vi "ReleaseBufferAndRemove.vi"(7 "index":i32, 8 "error in (no error)":errorcluster, 9 "pointer":u64, 10 "Buffer Name":string, 11 "Buffers":T1[](array[typedef])) -> (0 "error out":errorcluster, 2 "output buffer":T1, 3 "output buffers":T1[](array[typedef]))   [LabVIEW 2016]
uses:
  private/vis/BufferStruct.ctl
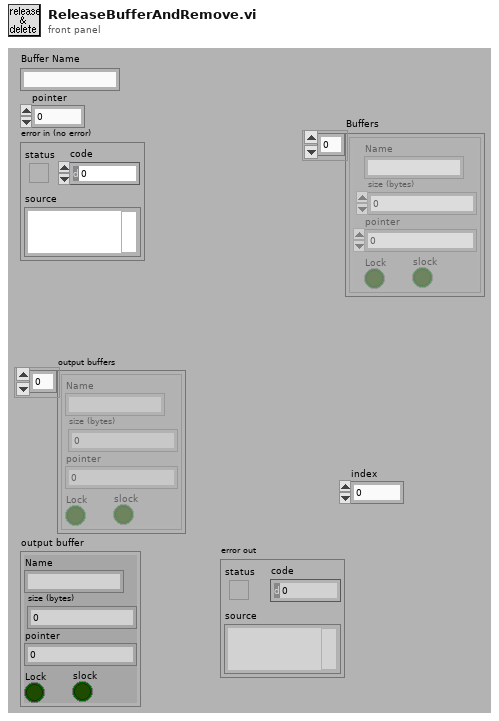
[diagram p1: front panel]
types:
  T1 = typedef "BufferStruct.ctl" = cluster{"Name":string, "size (bytes)":u64, "pointer":u64, "Lock":bool, "slock":bool}
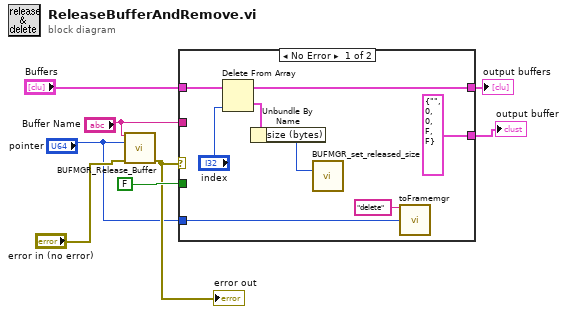
[diagram p0: block diagram]
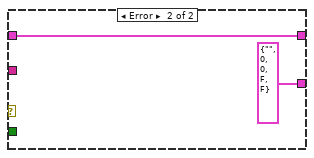
[diagram p2: hidden frame]
diagram:
  n1 = call "BUFMGR_Release_Buffer.vi"("Buffer Name"="Buffer Name", "buffer in"="pointer", "error in (no error)"="error in (no error)") -> ("error out"=w3:errorcluster)  [unwired: 12 out]
  "error out" <- w3
  n2 = case shown="No Error" w3 {
    tunnel: "Buffer Name" -> [_ _]
    tunnel: FALSE -> [_ _]
    tunnel: [w14 w18] -> w7
    tunnel: "Buffers" -> [w16 w18]
    tunnel: "pointer" -> [w10 _]
    tunnel: [T1 {"Name"="", "size (bytes)"=0, "pointer"=0, "Lock"=FALSE, "slock"=FALSE} ("output buffer") T1 {"Name"="", "size (bytes)"=0, "pointer"=0, "Lock"=FALSE, "slock"=FALSE} ("output buffer")] -> w1
    frame No Error {
      n3 = Delete From Array(array=w16, index="index") -> (deleted portion=w13:T1, array with subset deleted=w14:T1[])  [unwired: 1 in]
      n4 = Unbundle By Name(w13) -> ("size (bytes)"=w12:u64)
      n5 = call "BUFMGR_set_released_size.vi"("size in"=w12) -> ()  [unwired: 1 in, 14 out]
      n6 = call "toFramemgr.vi"("command"="delete", "bufpointer"=w10) -> ()  [unwired: 7 in, 7 out]
    }
    frame Error {
    }
  }
  "output buffers" <- w7
  "output buffer" <- w1
